vi "Strain Measurement Loop.vi"(6 "Which Program?":T1, 8 "error in":errorcluster, 9 "IBM OptoElectroMechanics Configuration":T2={"Parameter Analizer"={"Parameter Analyzer VISA Session"="COM1", "Sweeping Time Parameters"={"Integration Time"=0, "Short Integration Time (s)"=1.0, "Long Integration Time (s)"=0.0, "Wait Time Parameter"=1.0}, "Acquisition Mode"=enum."Sweeping Mode", "Status Polling Time (ms)"=0, "Comment"="Test VI", "SMU 1 - Sweeping"={"Start / Offset"=0.0, "Stop / Ratio"=1.0, "Step \n(linear only)"=0.01, "Compliance"=0.1, "Power \nCompliance"=0.0, "Mode"=0, "Function"=0, "Sweep Mode"=FALSE}, "SMU 2 - Sweeping"={"Start / Offset"=0.0, "Stop / Ratio"=1.0, "Step \n(linear only)"=0.01, "Compliance"=0.1, "Power \nCompliance"=0.0, "Mode"=0, "Function"=0, "Sweep Mode"=FALSE}, "SMU 3 - Sweeping"={"Start / Offset"=0.0, "Stop / Ratio"=1.0, "Step \n(linear only)"=0.01, "Compliance"=0.1, "Power \nCompliance"=0.0, "Mode"=0, "Function"=0, "Sweep Mode"=FALSE}, "SMU 4 - Sweeping"={"Start / Offset"=0.0, "Stop / Ratio"=1.0, "Step \n(linear only)"=0.01, "Compliance"=0.1, "Power \nCompliance"=0.0, "Mode"=0, "Function"=0, "Sweep Mode"=FALSE}, "Sweep Spacing"=0, "Range"=0, "SMU1 - Sampling"={"Source"=10.0, "Compliance"=1e-05, "Mode"=0, "Function"=FALSE}, "SMU2 - Sampling"={"Source"=1.0, "Compliance"=1.0, "Mode"=0, "Function"=FALSE}, "SMU3 - Sampling"={"Source"=10.0, "Compliance"=1e-05, "Mode"=0, "Function"=FALSE}, "SMU4 - Sampling"={"Source"=0.1, "Compliance"=60.0, "Mode"=10, "Function"=FALSE}, "Sampling Time Parameters"={"Initial Interval (s)"=0.1, "Number of Samples"=60, "Total Sampling Time (s)"=10.0, "Hold Time (s)"=0.0, "Sampling Mode"=0, "Sampling Time"=0}, "Stop Condition"={"Enable Delay (s)"=0.0, "Name"="", "Threshold"=0.0, "num. of events"=1, "Event"=0, "Stop Condition Enable"=FALSE}}, "Switching Matrix"={"Switching Matrix VISA Session"="GPIB0::18::INSTR", "Connections"=[{"Connections"=[FALSE, FALSE, FALSE, FALSE, FALSE, FALSE, FALSE, FALSE, FALSE, FALSE, FALSE, FALSE], "Connection Type"=enum."Disconnected"}, {"Connections"=[FALSE, FALSE, FALSE, FALSE, FALSE, FALSE, FALSE, FALSE, FALSE, FALSE, FALSE, FALSE], "Connection Type"=enum."Disconnected"}, {"Connections"=[FALSE, FALSE, FALSE, FALSE, FALSE, FALSE, FALSE, FALSE, FALSE, FALSE, FALSE, FALSE], "Connection Type"=enum."Disconnected"}, {"Connections"=[FALSE, FALSE, FALSE, FALSE, FALSE, FALSE, FALSE, FALSE, FALSE, FALSE, FALSE, FALSE], "Connection Type"=enum."Disconnected"}, {"Connections"=[FALSE, FALSE, FALSE, FALSE, FALSE, FALSE, FALSE, FALSE, FALSE, FALSE, FALSE, FALSE], "Connection Type"=enum."Disconnected"}, {"Connections"=[FALSE, FALSE, FALSE, FALSE, FALSE, FALSE, FALSE, FALSE, FALSE, FALSE, FALSE, FALSE], "Connection Type"=enum."Disconnected"}, {"Connections"=[FALSE, FALSE, FALSE, FALSE, FALSE, FALSE, FALSE, FALSE, FALSE, FALSE, FALSE, FALSE], "Connection Type"=enum."Disconnected"}, {"Connections"=[FALSE, FALSE, FALSE, FALSE, FALSE, FALSE, FALSE, FALSE, FALSE, FALSE, FALSE, FALSE], "Connection Type"=enum."Disconnected"}]}, "Stress Control"={"Stress Control VISA Session"="StrainMotor", "Axis"=0, "Motion"=0, "Destination (°)"=0.0, "Speed (°/s)"=4.0, "Position (°)"=25.0}, "Optical Spectrometer"={"Laser Settings"={"Laser Wavelength"=enum."365 nm", "Neutral Density Filter"=enum."100%"}, "Spectrometer Settings"={"Confocal Hole Size (µm)"=0.0, "Grating"=2, "Detector"=enum."InGaAs Array"}, "Acquisition Settings"={"Acquisition Mode"=enum."Multi-Window", "Spectal Position (nm)"=632.0, "From (nm)"=735.0, "To (nm)"=0.0, "Integration Time (s)"=0.0, "Number of Accumulations"=3, "AutoScanning"=FALSE, "Spike Removal"=FALSE}, "Path"=path "C:/07 - Prizes and Awards/Marie Curie Prize/Reply Editors Final NCOMMS(10).docx"}, "Switches & Mirrors"={"Relay VISA Session"="COM1", "Switches"={"Laser"=FALSE, "Video"=FALSE}, "Delays (ms)"={"Laser"=500, "Video"=1500}}, "Camera"={"Settings"={"Pixel clock"=20, "Frame rate"=30.0, "Exposure time"=33.21525, "Master Gain"=0, "Red Gain"=0, "Green Gain"=0, "Blue Gain"=0, "Auto Gain"=FALSE, "White-balance"=FALSE, "Color Correction"=FALSE}}, "XYZ Stage"={"Connection Settings"={"Tango VISA"="", "Baudrate"=57600, "Show Protocol?"=FALSE}, "Manual Control"={"North"=FALSE, "South"=FALSE, "West"=FALSE, "East"=FALSE, "Up"=FALSE, "Down"=FALSE, "Stop"=FALSE, "XY Step"=0.0, "Z step"=0.0}, "Coordinate Control"={"Motion Mode"=enum."Absolute", "Destination [mm]"=[]}}, "AutoFocus"={"Matching Criteria"={"Minimum Score"=700.0, "Color Score Weight"=700.0, "Minimum Contrast"=50, "Match Mode"=0, "Match Feature Mode"=0, "Subpixel Accuracy"=TRUE, "Color Sensitivity"=1, "Search Strategy"=1}, "Z Scan Parameters"={"Z Range"=1380.0, "Resolution"=5000.0, "Initial Direction"=enum."Up", "Focus Threshold"=0.1, "Ascent Constant"=0.1}, "Displacement"=0.0, "Transformation Matrix"=[]}, "Sava Data"={"Workspace Info"={"Device Name"="ProberHead_Tst_C29K3_7(2)", "Device Info"="ProberHead_Tst_C29", "Path"=path "C:/Users/gio/Desktop/ProbeHeadTest"}, "Instrument Configuration"={"Instrument"=enum."Unknown Instrument", "Configuration"="Test Configuration"}, "Stress Motor Position"=0.0, "Electrical Measurement"={"Sequence"=[], "V1"=[], "V2"=[], "V3"=[], "V4"=[], "I1"=[], "I2"=[], "I3"=[], "I4"=[]}, "Optical Spectrum"={"Intensity"=[], "Wavelength"=[], "Energy"=[], "Raman Shift"=[], "Detector Temperature"=0.0}}, "PlotData"={"Sliders"={"Strain Sequence"=0, "Instrument Sequence"=0}, "Measurement"={"Which Instrument?"=enum."No Plot", "Electrical Measurement"={"Sequence"=[], "V1"=[], "V2"=[], "V3"=[], "V4"=[], "I1"=[], "I2"=[], "I3"=[], "I4"=[]}, "Measurement Mode"=enum."Sweeping Mode", "Optical Spectrum"={"Intensity"=[], "Wavelength"=[], "Energy"=[], "Raman Shift"=[], "Detector Temperature"=0.0}}, "Instrument Steps"=[], "Strain Points"=[]}, "Instrument Sequence"={"Caller VI"=enum."User"}, "Strain Measurement"={"Stress Sequence "={"Max Motor Position"=1380.0, "# Intermediate Points"=5000, "Initial Direction"=enum."Tension"}, "Track?"=FALSE}} {"AutoFocus"."Displacement" scale=1.0..1000.0; "AutoFocus"."Z Scan Parameters"."Focus Threshold" min=0.0 max=1000.0 step=1.0 format="%#_2f"; "AutoFocus"."Z Scan Parameters"."Ascent Constant" min=0.0 max=1000.0 step=1.0 format="%#_2f"; "AutoFocus"."Z Scan Parameters"."Resolution" min=0.0 max=1.0 step=0.01 format="%_2g"; "AutoFocus"."Z Scan Parameters"."Z Range" format="%_3g"; "AutoFocus"."Matching Criteria"."Match Mode" items=["Shift Invariant", "Rotation Invariant"]; "AutoFocus"."Matching Criteria"."Match Feature Mode" items=["Color and Shape", "Color", "Shape"]; "AutoFocus"."Matching Criteria"."Color Sensitivity" items=["Low Sensitivity", "Medium Sensitivity", "High Sensitivity"]; "AutoFocus"."Matching Criteria"."Search Strategy" items=["Conservative", "Balance", "Aggressive", "Very Aggressive"]; "XYZ Stage"."Manual Control"."Z step" scale=0.1..10.0; "XYZ Stage"."Manual Control"."XY Step" scale=0.1..1000.0; "Camera"."Settings"."Blue Gain" min=0 max=100 scale=0.0..100.0; "Camera"."Settings"."Green Gain" min=0 max=100 scale=0.0..100.0; "Camera"."Settings"."Red Gain" min=0 max=100 scale=0.0..100.0; "Camera"."Settings"."Master Gain" min=0 max=100 scale=0.0..100.0; "Camera"."Settings"."Exposure time" min=0.101625 max=159.246375 step=0.101625 scale=0.101625..159.246375 scale format="%#.3g"; "Camera"."Settings"."Frame rate" min=2.7455631699174137 max=6.2675785993528725 step=0.000101625 scale=2.7455631699174137..6.2675785993528725 scale format="%^#_3g"; "Camera"."Settings"."Pixel clock" min=5 max=43 scale=5.0..43.0; "PlotData"."Sliders"."Instrument Sequence" scale=0.0..10.0; "PlotData"."Sliders"."Strain Sequence" scale=0.0..10.0; "Strain Measurement"."Stress Sequence"."# Intermediate Points" max=1390; "Parameter Analizer"."Stop Condition"."Event" items=["Value > Threshold", "Value < Threshold", "| Value | > | Threshold |", "| Value | < | Threshold |"]; "Parameter Analizer"."Stop Condition"."Threshold" format="%^.2e"; "Parameter Analizer"."Stop Condition"."Enable Delay (s)" format="%.1f"; "Parameter Analizer"."Sampling Time Parameters"."Sampling Time" items=["Auto (linear only)", "No Limit", "Set Limit"]; "Parameter Analizer"."Sampling Time Parameters"."Sampling Mode" items=["Linear", "Log10", "Log25", "Log50", "Thinned Out"]; "Parameter Analizer"."Sampling Time Parameters"."Hold Time (s)" format="%.4f"; "Parameter Analizer"."Sampling Time Parameters"."Total Sampling Time (s)" format="%.1f"; "Parameter Analizer"."Sampling Time Parameters"."Initial Interval (s)" format="%^.3e"; "Parameter Analizer"."SMU 4 - Sweeping"."Function" items=["Disabled", "Var 1", "Var 2", "Var 1'", "Constant"]; "Parameter Analizer"."SMU 4 - Sweeping"."Mode" items=["V", "I", "V pulse", "I  pulse", "Common"]; "Parameter Analizer"."SMU 4 - Sweeping"."Power \nCompliance" format="%^.2e"; "Parameter Analizer"."SMU 4 - Sweeping"."Compliance" format="%^.2e"; "Parameter Analizer"."SMU 4 - Sweeping"."Step \n(linear only)" format="%^.4e"; "Parameter Analizer"."SMU 4 - Sweeping"."Stop / Ratio" format="%^.4e"; "Parameter Analizer"."SMU 4 - Sweeping"."Start / Offset" format="%^.4e"; "Parameter Analizer"."SMU 3 - Sweeping"."Function" items=["Disabled", "Var 1", "Var 2", "Var 1'", "Constant"]; "Parameter Analizer"."SMU 3 - Sweeping"."Mode" items=["V", "I", "V pulse", "I  pulse", "Common"]; "Parameter Analizer"."SMU 3 - Sweeping"."Power \nCompliance" format="%^.2e"; "Parameter Analizer"."SMU 3 - Sweeping"."Compliance" format="%^.2e"; "Parameter Analizer"."SMU 3 - Sweeping"."Step \n(linear only)" format="%^.4e"; "Parameter Analizer"."SMU 3 - Sweeping"."Stop / Ratio" format="%^.4e"; "Parameter Analizer"."SMU 3 - Sweeping"."Start / Offset" format="%^.4e"; "Parameter Analizer"."SMU 2 - Sweeping"."Function" items=["Disabled", "Var 1", "Var 2", "Var 1'", "Constant"]; "Parameter Analizer"."SMU 2 - Sweeping"."Mode" items=["V", "I", "V pulse", "I  pulse", "Common"]; "Parameter Analizer"."SMU 2 - Sweeping"."Power \nCompliance" format="%^.2e"; "Parameter Analizer"."SMU 2 - Sweeping"."Compliance" format="%^.2e"; "Parameter Analizer"."SMU 2 - Sweeping"."Step \n(linear only)" format="%^.4e"; "Parameter Analizer"."SMU 2 - Sweeping"."Stop / Ratio" format="%^.4e"; "Parameter Analizer"."SMU 2 - Sweeping"."Start / Offset" format="%^.4e"; "Parameter Analizer"."SMU 1 - Sweeping"."Function" items=["Disabled", "Var 1", "Var 2", "Var 1'", "Constant"]; "Parameter Analizer"."SMU 1 - Sweeping"."Mode" items=["V", "I", "V pulse", "I  pulse", "Common"]; "Parameter Analizer"."SMU 1 - Sweeping"."Power \nCompliance" format="%^.2e"; "Parameter Analizer"."SMU 1 - Sweeping"."Compliance" format="%^.2e"; "Parameter Analizer"."SMU 1 - Sweeping"."Step \n(linear only)" format="%^.4e"; "Parameter Analizer"."SMU 1 - Sweeping"."Stop / Ratio" format="%^.4e"; "Parameter Analizer"."SMU 1 - Sweeping"."Start / Offset" format="%^.4e"; "Parameter Analizer"."Sweeping Time Parameters"."Long Integration Time (s)" scale=0.02..2.0; "Parameter Analizer"."Sweeping Time Parameters"."Short Integration Time (s)" scale=8e-05..0.00192; "Parameter Analizer"."Sweeping Time Parameters"."Integration Time" items=["Short", "Long"]; "Parameter Analizer"."Sweeping Time Parameters"."Wait Time Parameter" format="%.1f"; "Parameter Analizer"."SMU4 - Sampling"."Mode" items=["V", "I", "Common"]; "Parameter Analizer"."SMU4 - Sampling"."Compliance" format="%^.2e"; "Parameter Analizer"."SMU4 - Sampling"."Source" format="%^.3e"; "Parameter Analizer"."SMU3 - Sampling"."Mode" items=["V", "I", "Common"]; "Parameter Analizer"."SMU3 - Sampling"."Compliance" format="%^.2e"; "Parameter Analizer"."SMU3 - Sampling"."Source" format="%^.3e"; "Parameter Analizer"."SMU2 - Sampling"."Mode" items=["V", "I", "Common"]; "Parameter Analizer"."SMU2 - Sampling"."Compliance" format="%^.2e"; "Parameter Analizer"."SMU2 - Sampling"."Source" format="%^.3e"; "Parameter Analizer"."SMU1 - Sampling"."Mode" items=["V", "I", "Common"]; "Parameter Analizer"."SMU1 - Sampling"."Compliance" format="%^.2e"; "Parameter Analizer"."SMU1 - Sampling"."Source" format="%^.3e"; "Parameter Analizer"."Range" items=["auto", "fixed", "limited"]; "Parameter Analizer"."Sweep Spacing" items=["linear", "log 10", "log 25", "log 50"]; "Stress Control"."Axis" min=1 max=3; "Stress Control"."Position (°)" format="%.6g"; "Stress Control"."Speed (°/s)" min=0.0 max=4.0 format="%.6f"; "Stress Control"."Destination (°)" min=-2000000000.0 max=2000000000.0 format="%.6f"; "Stress Control"."Motion" items=["Absolute", "Relative"]; "Optical Spectrometer"."Spectrometer Settings"."Grating" items=["1800 l/mm", "150 l/mm"]}, 10 "Message Queues out":T58, 11 "Notifiers":T45) -> (0 "error out":errorcluster)   [LabVIEW 2014]
uses:
  support/Message Queue/All Message Queues.ctl
  support/Message Queue/Message Cluster.ctl
  support/Notifiers/Notifiers.ctl
  support/Message Handler Loop Notifiers.ctl
  Hardware Control/Parameter Analyzer/Parameter Analyzer Notifiers.ctl
  Hardware Control/Switching Matrix/Switching Matrix Notifiers.ctl
  Hardware Control/Stress Control/StressControl Notifiers.ctl
  Hardware Control/Spectrometer/Spectrometer Notifiers.ctl
  Hardware Control/Switches and Mirrors/SwitchesMirrors Notifiers.ctl
  Hardware Control/Camera/Camera Notifiers.ctl
  Hardware Control/XYZ Stage/XYZ Notifications.ctl
  Hardware Control/Autofocus/Autofocus Notifiers.ctl
  Measurements/Optoelectronic Measurement/Optoelectronic Notifiers.ctl
  Measurements/Save Data/SaveData Notifiers.ctl
  Measurements/Instrument Sequence/Instrument Sequence Notifiers.ctl
  support/Configuration/Configuration.ctl
  Hardware Control/Parameter Analyzer/Parameter Analyzer Config.ctl
  Hardware Control/Parameter Analyzer/Parameter Analyzer Integration Parameters.ctl
  Hardware Control/Parameter Analyzer/Parameter Analyzer SMU Sweeping.ctl
  Hardware Control/Parameter Analyzer/Parameter Analyzer Sweep Spacing.ctl
  Hardware Control/Parameter Analyzer/Parameter Analyzer SMU Range.ctl
  Hardware Control/Parameter Analyzer/Parameter Analyzer SMU Sampling.ctl
  Hardware Control/Parameter Analyzer/Parameter Analyzer Sampling Parameters.ctl
  Hardware Control/Parameter Analyzer/Parameter Analyzer Stop Sampling Conditions.ctl
  Hardware Control/Switching Matrix/Switching Matrix Config.ctl
  Hardware Control/Stress Control/StressControl Config.ctl
  Hardware Control/Spectrometer/Spectrometer Config.ctl
  Hardware Control/Spectrometer/Laser Settings.ctl
  Hardware Control/Spectrometer/Laser.ctl
  Hardware Control/Spectrometer/Filter.ctl
  Hardware Control/Spectrometer/Grating Detector Settings.ctl
  Hardware Control/Spectrometer/Grating.ctl
  Hardware Control/Spectrometer/Detector.ctl
  Hardware Control/Spectrometer/Acquisition Settings.ctl
  Hardware Control/Switches and Mirrors/SwitchesMirrors Config.ctl
  Hardware Control/Switches and Mirrors/SwitchesMirrors Status.ctl
  Hardware Control/Camera/Camera Config.ctl
  Hardware Control/Camera/Camera Settings.ctl
  Hardware Control/XYZ Stage/XYZ Config.ctl
  Hardware Control/XYZ Stage/XYZ Connection Settings.ctl
  Hardware Control/XYZ Stage/XYZ Stage Control.ctl
  Hardware Control/XYZ Stage/XYZ Coordinate Control.ctl
  Hardware Control/Autofocus/AutoFocus Config.ctl
  Hardware Control/Autofocus/ZScan.ctl
  <vilib>/Analysis/Matrix/Datatypes/RealMatrix.ctl
  Measurements/Save Data/SaveData Config.ctl
  Measurements/Save Data/SaveData Workspace Info.ctl
  Measurements/Save Data/SaveData Instrument Configuration.ctl
  Measurements/Instrument Sequence/Instrument List.ctl
  Hardware Control/Spectrometer/Spectral Data.ctl
  Measurements/Plot Data/PlotData Config.ctl
  Measurements/Plot Data/Measurement.ctl
  Measurements/Plot Data/WhichInstrument.ctl
  Hardware Control/Parameter Analyzer/Electrical Data.ctl
  Measurements/Instrument Sequence/Instrument Steps.ctl
  Measurements/Instrument Sequence/Action.ctl
  Measurements/Instrument Sequence/Instrument Sequence Config.ctl
  Measurements/Strain Measurement/Strain Measurement Config.ctl
  Measurements/Instrument Sequence/Instrument Stequence - Which Program.ctl
  Measurements/Strain Measurement/Strain Measurement Function.ctl
  support/Message Queue/Message Queue.lvlib
  <vilib>/Analysis/Matrix/NI_Matrix.lvlib
panel:
  # "LICENSED MATERIALS – PROPERTY OF IBM\nCopyright IBM Corp. 2016,\nALL RIGHTS RESERVED"
  # "XY"
  # "Z"
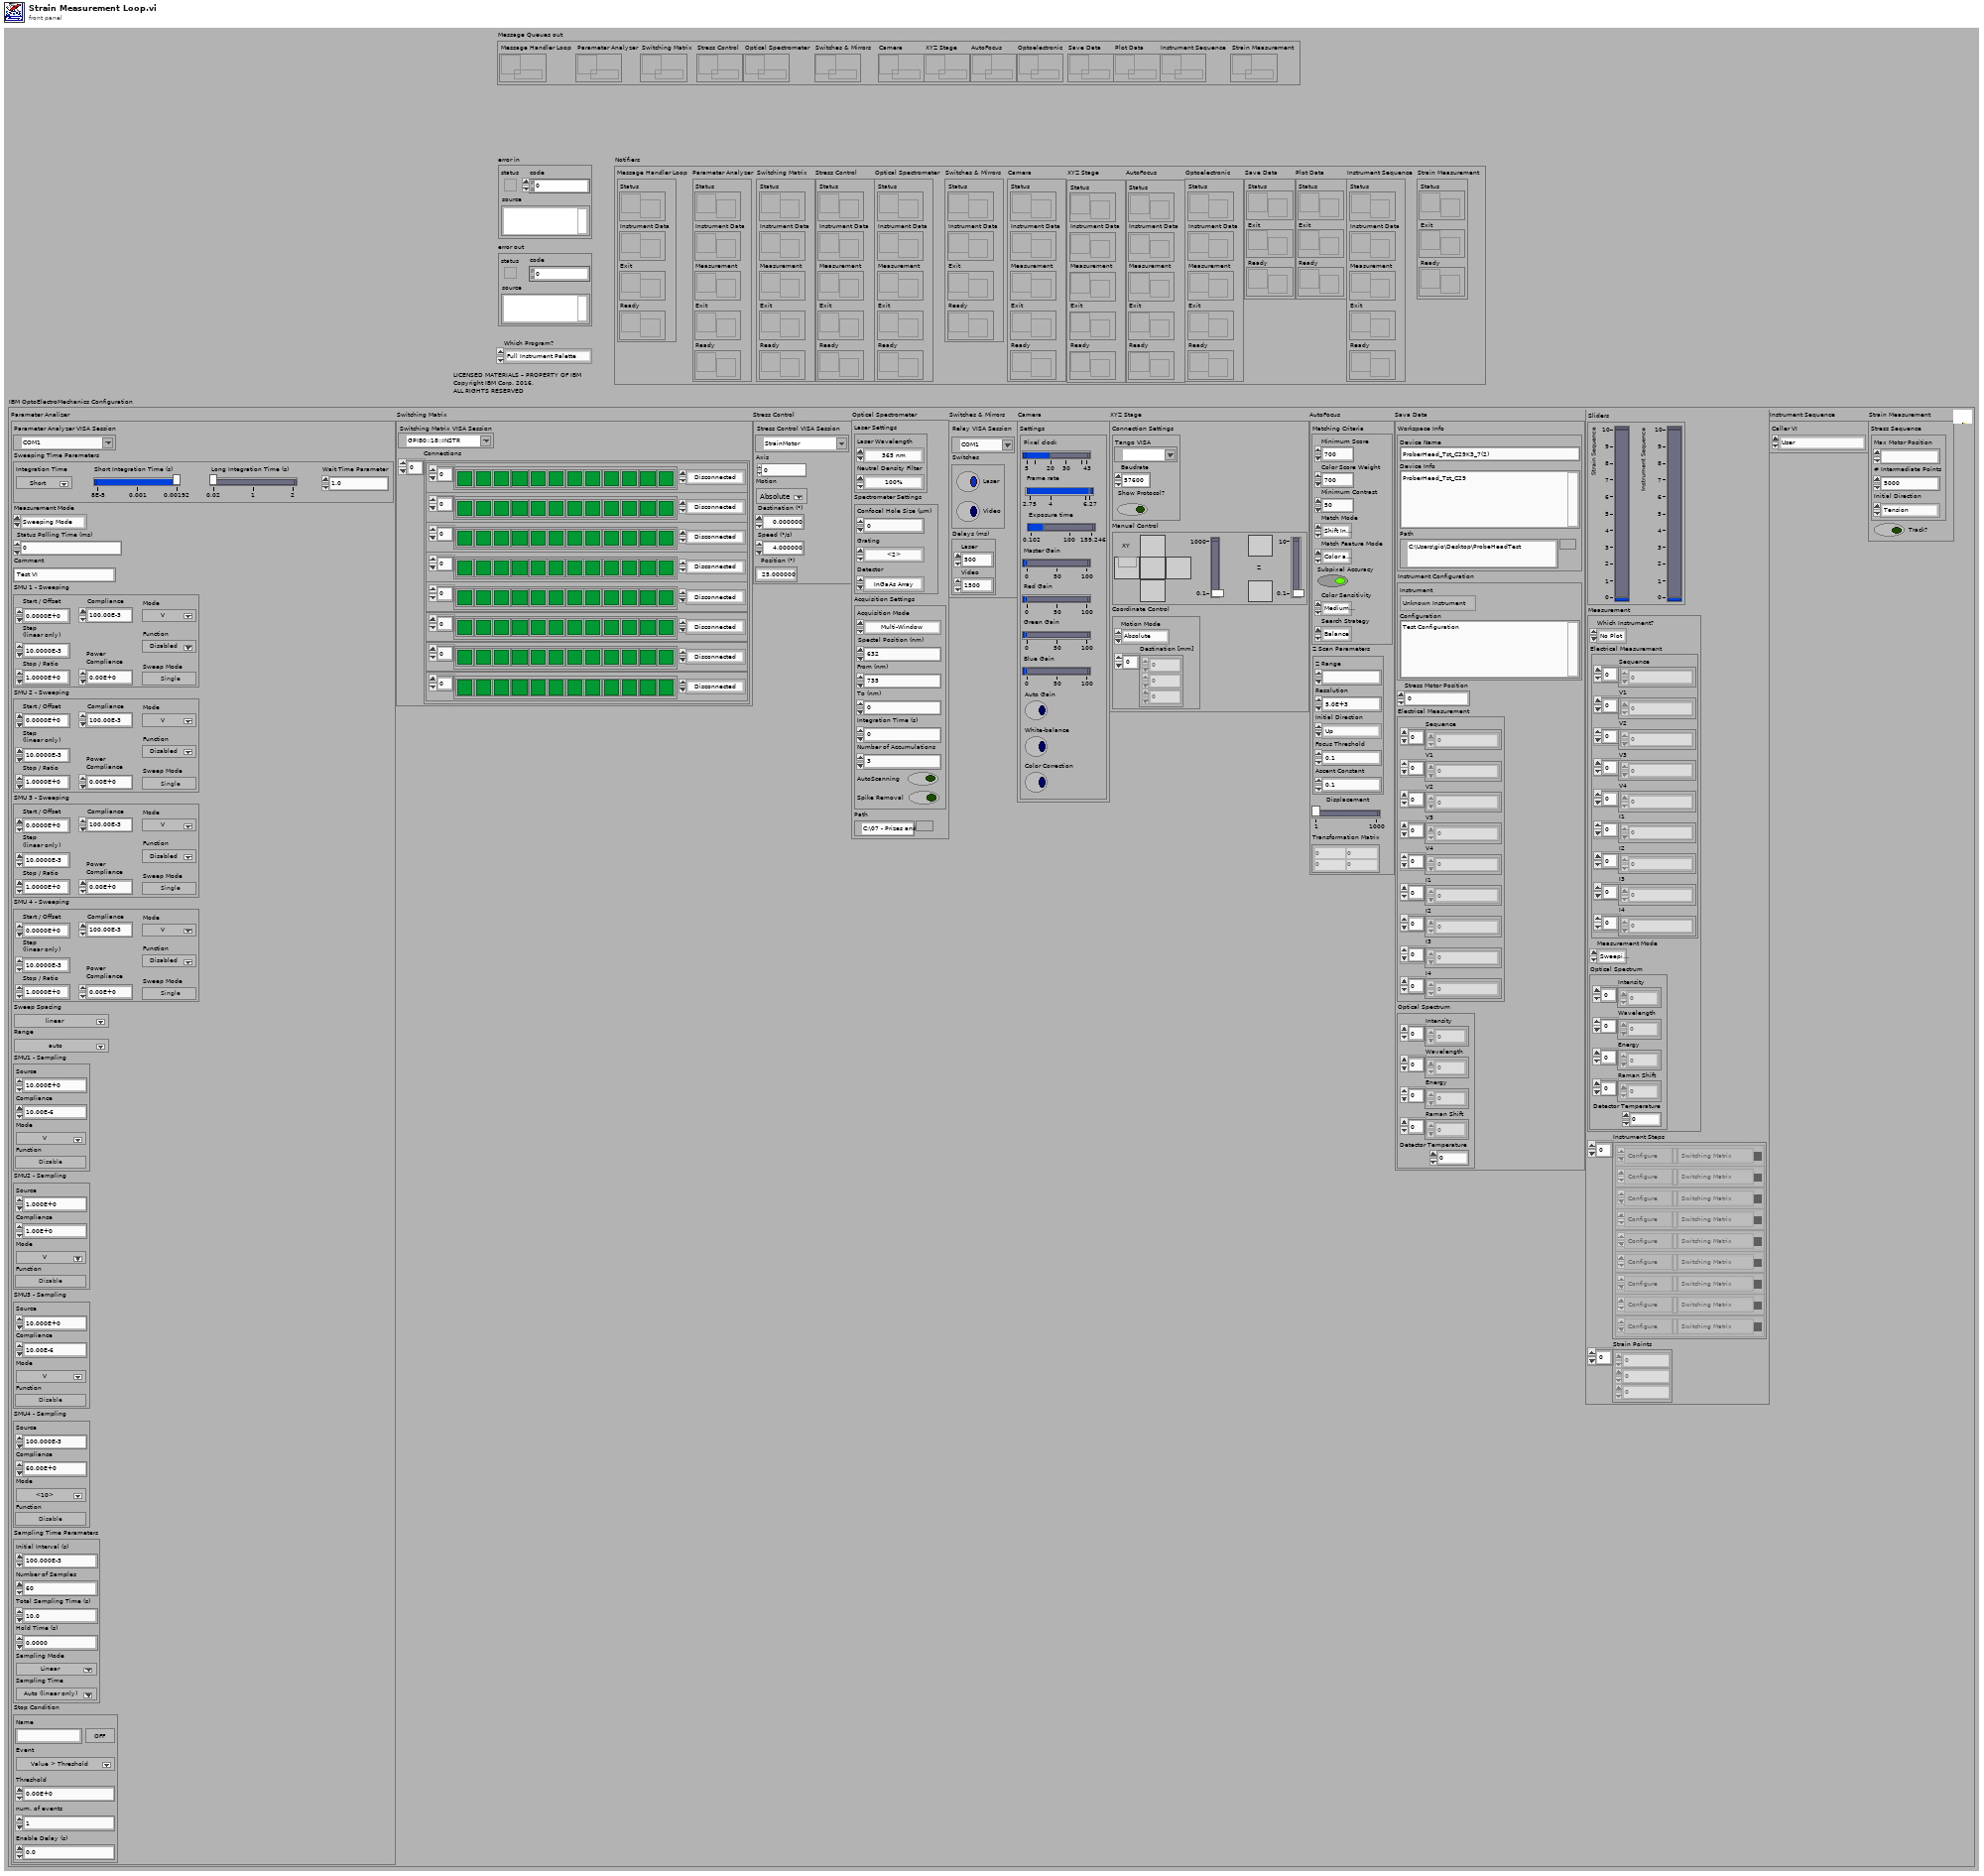
[diagram p1: front panel]
types:
  T1 = typedef "Instrument Stequence - Which Program.ctl" = enum16{"Full Instrument Palette", "Strain Electrical"}
  T2 = typedef "Configuration.ctl" = cluster{"Parameter Analizer":T3, "Switching Matrix":T11, "Stress Control":T12, "Optical Spectrometer":T13, "Switches & Mirrors":T21, "Camera":T23, "XYZ Stage":T25, "AutoFocus":T29, "Sava Data":T32, "PlotData":T37, "Instrument Sequence":T43, "Strain Measurement":T44}
  T3 = typedef "Parameter Analyzer Config.ctl" = cluster{"Parameter Analyzer VISA Session":refnum<visa-resource-name>, "Sweeping Time Parameters":T4, "Acquisition Mode":enum32{"Sweeping Mode", "Sampling Mode"}, "Status Polling Time (ms)":u32, "Comment":string, "SMU 1 - Sweeping":T5, "SMU 2 - Sweeping":T5, "SMU 3 - Sweeping":T5, "SMU 4 - Sweeping":T5, "Sweep Spacing":T6, "Range":T7, "SMU1 - Sampling":T8, "SMU2 - Sampling":T8, "SMU3 - Sampling":T8, "SMU4 - Sampling":T8, "Sampling Time Parameters":T9, "Stop Condition":T10}
  T4 = typedef "Parameter Analyzer Integration Parameters.ctl" = cluster{"Integration Time":u32, "Short Integration Time (s)":dbl, "Long Integration Time (s)":dbl, "Wait Time Parameter":dbl}
  T5 = typedef "Parameter Analyzer SMU Sweeping.ctl" = cluster{"Start / Offset":dbl, "Stop / Ratio":dbl, "Step \n(linear only)":dbl, "Compliance":dbl, "Power \nCompliance":dbl, "Mode":u32, "Function":i32, "Sweep Mode":bool}
  T6 = typedef "Parameter Analyzer Sweep Spacing.ctl" = u16
  T7 = typedef "Parameter Analyzer SMU Range.ctl" = u16
  T8 = typedef "Parameter Analyzer SMU Sampling.ctl" = cluster{"Source":dbl, "Compliance":dbl, "Mode":u32, "Function":bool}
  T9 = typedef "Parameter Analyzer Sampling Parameters.ctl" = cluster{"Initial Interval (s)":dbl, "Number of Samples":i32, "Total Sampling Time (s)":dbl, "Hold Time (s)":dbl, "Sampling Mode":i32, "Sampling Time":i32}
  T10 = typedef "Parameter Analyzer Stop Sampling Conditions.ctl" = cluster{"Enable Delay (s)":dbl, "Name":string, "Threshold":dbl, "num. of events":i32, "Event":i32, "Stop Condition Enable":bool}
  T11 = typedef "Switching Matrix Config.ctl" = cluster{"Switching Matrix VISA Session":refnum<visa-resource-name>, "Connections":cluster{"Connections":bool[], "Connection Type":enum16{"Disconnected", "Make - Break", "Break - Make"}}[]}
  T12 = typedef "StressControl Config.ctl" = cluster{"Stress Control VISA Session":refnum<visa-resource-name>, "Axis":i32, "Motion":u16, "Destination (°)":dbl, "Speed (°/s)":dbl, "Position (°)":dbl}
  T13 = typedef "Spectrometer Config.ctl" = cluster{"Laser Settings":T14, "Spectrometer Settings":T17, "Acquisition Settings":T20, "Path":path}
  T14 = typedef "Laser Settings.ctl" = cluster{"Laser Wavelength":T15, "Neutral Density Filter":T16}
  T15 = typedef "Laser.ctl" = enum16{"633 nm", "784 nm", "532 nm", "365 nm"}
  T16 = typedef "Filter.ctl" = enum16{"100%", "50%", "25%", "10%", "1%", "0.1%", "0.01%"}
  T17 = typedef "Grating Detector Settings.ctl" = cluster{"Confocal Hole Size (µm)":dbl, "Grating":T18, "Detector":T19}
  T18 = typedef "Grating.ctl" = u16
  T19 = typedef "Detector.ctl" = enum16{"InGaAs Array", "Silicon CCD"}
  T20 = typedef "Acquisition Settings.ctl" = cluster{"Acquisition Mode":enum16{"Single Window", "Multi-Window"}, "Spectal Position (nm)":dbl, "From (nm)":dbl, "To (nm)":dbl, "Integration Time (s)":dbl, "Number of Accumulations":i32, "AutoScanning":bool, "Spike Removal":bool}
  T21 = typedef "SwitchesMirrors Config.ctl" = cluster{"Relay VISA Session":refnum<visa-resource-name>, "Switches":T22, "Delays (ms)":cluster{"Laser":u32, "Video":u32}}
  T22 = typedef "SwitchesMirrors Status.ctl" = cluster{"Laser":bool, "Video":bool}
  T23 = typedef "Camera Config.ctl" = cluster{"Settings":T24}
  T24 = typedef "Camera Settings.ctl" = cluster{"Pixel clock":i32, "Frame rate":dbl, "Exposure time":dbl, "Master Gain":i32, "Red Gain":i32, "Green Gain":i32, "Blue Gain":i32, "Auto Gain":bool, "White-balance":bool, "Color Correction":bool}
  T25 = typedef "XYZ Config.ctl" = cluster{"Connection Settings":T26, "Manual Control":T27, "Coordinate Control":T28}
  T26 = typedef "XYZ Connection Settings.ctl" = cluster{"Tango VISA":refnum<visa-resource-name>, "Baudrate":i32, "Show Protocol?":bool}
  T27 = typedef "XYZ Stage Control.ctl" = cluster{"North":bool, "South":bool, "West":bool, "East":bool, "Up":bool, "Down":bool, "Stop":bool, "XY Step":dbl, "Z step":dbl}
  T28 = typedef "XYZ Coordinate Control.ctl" = cluster{"Motion Mode":enum16{"Absolute", "Relative"}, "Destination [mm]":dbl[]}
  T29 = typedef "AutoFocus Config.ctl" = cluster{"Matching Criteria":cluster{"Minimum Score":sgl, "Color Score Weight":sgl, "Minimum Contrast":i32, "Match Mode":u32, "Match Feature Mode":u32, "Subpixel Accuracy":bool, "Color Sensitivity":u32, "Search Strategy":u32}, "Z Scan Parameters":T30, "Displacement":dbl, "Transformation Matrix":T31}
  T30 = typedef "ZScan.ctl" = cluster{"Z Range":ext, "Resolution":dbl, "Initial Direction":enum16{"Up", "Down"}, "Focus Threshold":dbl, "Ascent Constant":dbl}
  T31 = typedef "NI_Matrix.lvlib/RealMatrix.ctl" = dbl[][]
  T32 = typedef "SaveData Config.ctl" = cluster{"Workspace Info":T33, "Instrument Configuration":T34, "Stress Motor Position":dbl, "Electrical Measurement":cluster{"Sequence":dbl[], "V1":dbl[], "V2":dbl[], "V3":dbl[], "V4":dbl[], "I1":dbl[], "I2":dbl[], "I3":dbl[], "I4":dbl[]}, "Optical Spectrum":T36}
  T33 = typedef "SaveData Workspace Info.ctl" = cluster{"Device Name":string, "Device Info":string, "Path":path}
  T34 = typedef "SaveData Instrument Configuration.ctl" = cluster{"Instrument":T35, "Configuration":string}
  T35 = typedef "Instrument List.ctl" = enum32{"Unknown Instrument", "Switching Matrix", "Parameter Analyzer", "Optical Spectrometer", "Optoelectronic", "Autofocus"}
  T36 = typedef "Spectral Data.ctl" = cluster{"Intensity":dbl[], "Wavelength":dbl[], "Energy":dbl[], "Raman Shift":dbl[], "Detector Temperature":dbl}
  T37 = typedef "PlotData Config.ctl" = cluster{"Sliders":cluster{"Strain Sequence":i32, "Instrument Sequence":i32}, "Measurement":T38, "Instrument Steps":T41, "Strain Points":dbl[]}
  T38 = typedef "Measurement.ctl" = cluster{"Which Instrument?":T39, "Electrical Measurement":T40, "Measurement Mode":enum16{"Sweeping Mode", "Sampling Mode"}, "Optical Spectrum":T36}
  T39 = typedef "WhichInstrument.ctl" = enum16{"No Plot", "Spectrometer", "Parameter Analyzer", "Optoelectronic"}
  T40 = typedef "Electrical Data.ctl" = cluster{"Sequence":dbl[], "V1":dbl[], "V2":dbl[], "V3":dbl[], "V4":dbl[], "I1":dbl[], "I2":dbl[], "I3":dbl[], "I4":dbl[]}
  T41 = typedef "Instrument Steps.ctl" = cluster{"Action":T42, "Configuration":variant, "Instrument":T35, "Status":enum8{"False", "True", "Mixed"}}[]
  T42 = typedef "Action.ctl" = enum32{"Configure", "Measure"}
  T43 = typedef "Instrument Sequence Config.ctl" = cluster{"Caller VI":enum16{"User", "Stress Measurement VI"}}
  T44 = typedef "Strain Measurement Config.ctl" = cluster{"Stress Sequence ":cluster{"Max Motor Position":ext, "# Intermediate Points":u32, "Initial Direction":enum16{"Tension", "Compression"}}, "Track?":bool}
  T45 = typedef "Notifiers.ctl" = cluster{"Message Handler Loop":T46, "Parameter Analyzer":T47, "Switching Matrix":T48, "Stress Control":T49, "Optical Spectrometer":T50, "Switches & Mirrors":T51, "Camera":T52, "XYZ Stage":T53, "AutoFocus":T54, "Optoelectronic":T55, "Save Data":T56, "Plot Data":T56, "Instrument Sequence":T57, "Strain Measurement":cluster{"Status":refnum<notifier>, "Exit":refnum<notifier>, "Ready":refnum<notifier>}}
  T46 = typedef "Message Handler Loop Notifiers.ctl" = cluster{"Status":refnum<notifier>, "Instrument Data":refnum<notifier>, "Exit":refnum<notifier>, "Ready":refnum<notifier>}
  T47 = typedef "Parameter Analyzer Notifiers.ctl" = cluster{"Status":refnum<notifier>, "Instrument Data":refnum<notifier>, "Measurement":refnum<notifier>, "Exit":refnum<notifier>, "Ready":refnum<notifier>}
  T48 = typedef "Switching Matrix Notifiers.ctl" = cluster{"Status":refnum<notifier>, "Instrument Data":refnum<notifier>, "Measurement":refnum<notifier>, "Exit":refnum<notifier>, "Ready":refnum<notifier>}
  T49 = typedef "StressControl Notifiers.ctl" = cluster{"Status":refnum<notifier>, "Instrument Data":refnum<notifier>, "Measurement":refnum<notifier>, "Exit":refnum<notifier>, "Ready":refnum<notifier>}
  T50 = typedef "Spectrometer Notifiers.ctl" = cluster{"Status":refnum<notifier>, "Instrument Data":refnum<notifier>, "Measurement":refnum<notifier>, "Exit":refnum<notifier>, "Ready":refnum<notifier>}
  T51 = typedef "SwitchesMirrors Notifiers.ctl" = cluster{"Status":refnum<notifier>, "Instrument Data":refnum<notifier>, "Exit":refnum<notifier>, "Ready":refnum<notifier>}
  T52 = typedef "Camera Notifiers.ctl" = cluster{"Status":refnum<notifier>, "Instrument Data":refnum<notifier>, "Measurement":refnum<notifier>, "Exit":refnum<notifier>, "Ready":refnum<notifier>}
  T53 = typedef "XYZ Notifications.ctl" = cluster{"Status":refnum<notifier>, "Instrument Data":refnum<notifier>, "Measurement":refnum<notifier>, "Exit":refnum<notifier>, "Ready":refnum<notifier>}
  T54 = typedef "Autofocus Notifiers.ctl" = cluster{"Status":refnum<notifier>, "Instrument Data":refnum<notifier>, "Measurement":refnum<notifier>, "Exit":refnum<notifier>, "Ready":refnum<notifier>}
  T55 = typedef "Optoelectronic Notifiers.ctl" = cluster{"Status":refnum<notifier>, "Instrument Data":refnum<notifier>, "Measurement":refnum<notifier>, "Exit":refnum<notifier>, "Ready":refnum<notifier>}
  T56 = typedef "SaveData Notifiers.ctl" = cluster{"Status":refnum<notifier>, "Exit":refnum<notifier>, "Ready":refnum<notifier>}
  T57 = typedef "Instrument Sequence Notifiers.ctl" = cluster{"Status":refnum<notifier>, "Instrument Data":refnum<notifier>, "Measurement":refnum<notifier>, "Exit":refnum<notifier>, "Ready":refnum<notifier>}
  T58 = typedef "Message Queue.lvlib/All Message Queues.ctl" = cluster{"Message Handler Loop":refnum<queue>, "Parameter Analyzer":refnum<queue>, "Switching Matrix":refnum<queue>, "Stress Control":refnum<queue>, "Optical Spectrometer":refnum<queue>, "Switches & Mirrors":refnum<queue>, "Camera":refnum<queue>, "XYZ Stage":refnum<queue>, "AutoFocus":refnum<queue>, "Optoelectronic":refnum<queue>, "Save Data":refnum<queue>, "Plot Data":refnum<queue>, "Instrument Sequence":refnum<queue>, "Strain Measurement":refnum<queue>}
  T59 = typedef "Strain Measurement Data.ctl" = cluster{"Configuration":T44, "Refnums":T60}
  T60 = typedef "Strain Measurement Refnums.ctl" = cluster{"Instrument Steps":refnum<vi>, "Sequence Progress":refnum<vi>, "Device ID":refnum<vi>, "Device Information":refnum<vi>, "Pause-Resume":refnum<vi>, "Track":refnum<vi>, "Plot":T61}
  T61 = typedef "Electrical Data Plot Refnums.ctl" = cluster{"Plot List":refnum<vi>, "Voltage Plot":refnum<vi>, "Current Plot":refnum<vi>, "IV Characteristic":refnum<vi>, "dI/dV-V Characteristic":refnum<vi>}
  T62 = typedef "Strain Measurement Function.ctl" = enum16{"Get Stress Controller Status", "Define Strain Sequence", "Update Track", "Decide on Track", "Reset Strain Sequence", "Start Strain Measurement", "Set Strain Sequence Step", "Add Instrument Sequence Step", "Delete Instrument Sequence Step", "Clear Instrument Sequence", "Reset Instrument Sequence", "Load Instrument Sequence", "Save Instrument Sequence", "Measure Instrument Sequence", "Choose What Next", "Configure Stress Control", "Set Workspace Data", "Save to Workspace", "Update Sequence Status", "Pause", "Stop", "Update Refnums"}
  T63 = cluster{"Max Motor Position":ext, "# Intermediate Points":u32, "Initial Direction":enum16{"Tension", "Compression"}}
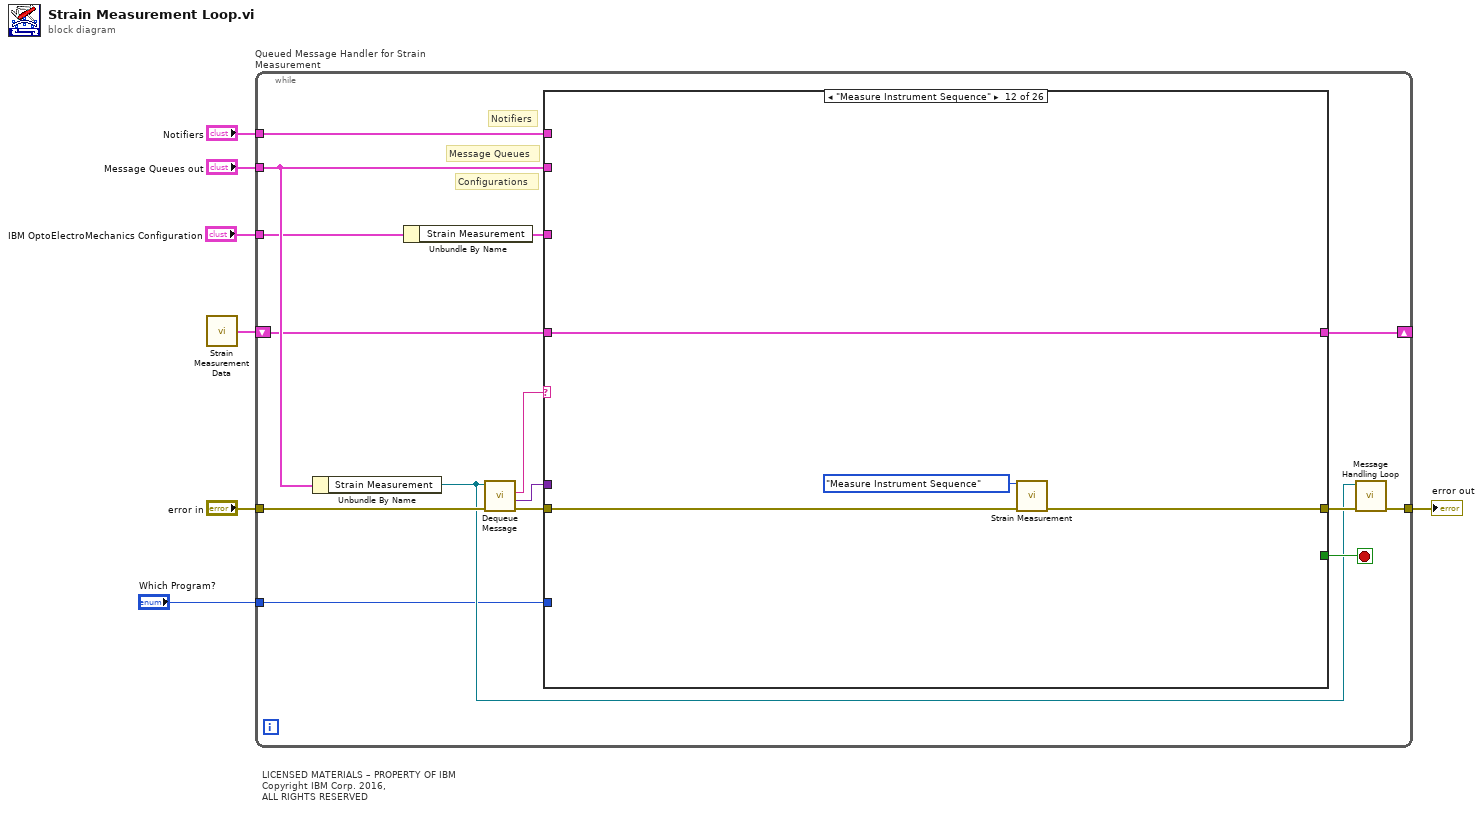
[diagram p0: block diagram]
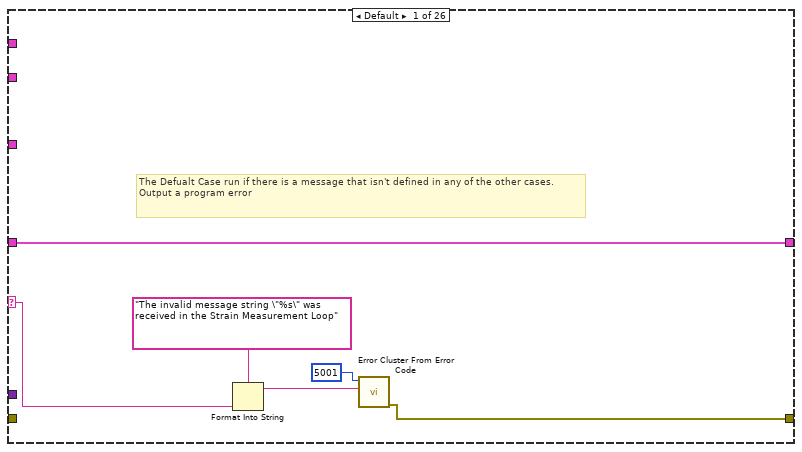
[diagram p2: hidden frame]
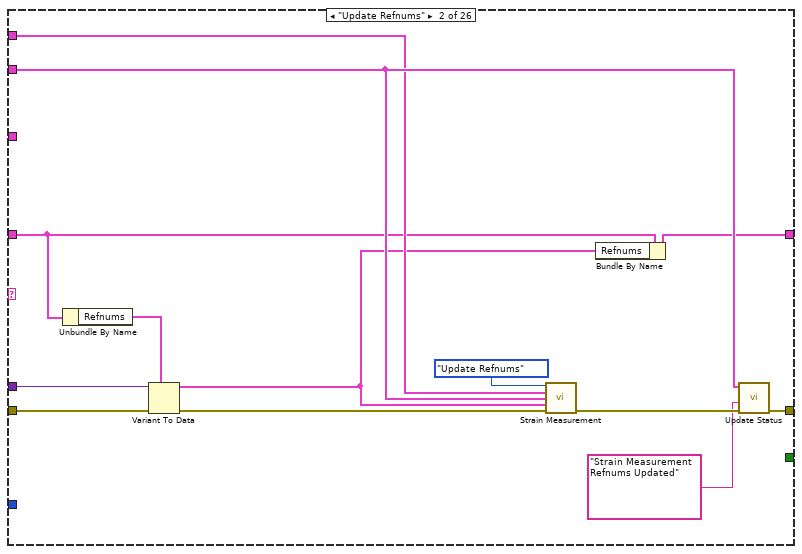
[diagram p3: hidden frame]
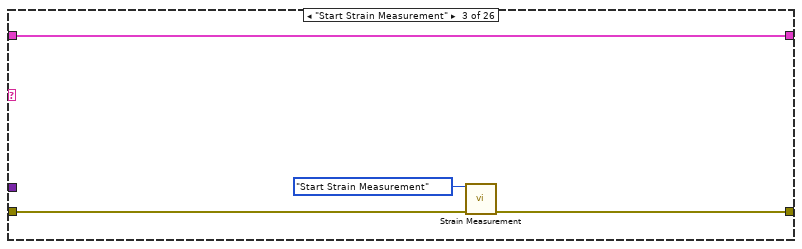
[diagram p4: hidden frame]
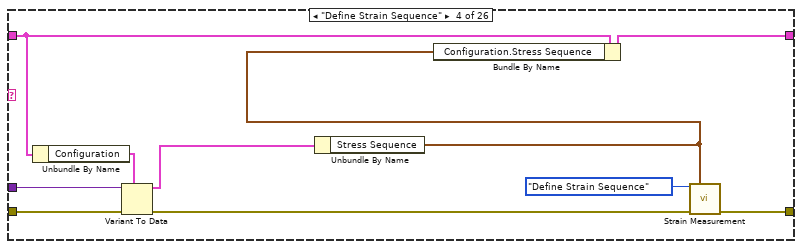
[diagram p5: hidden frame]
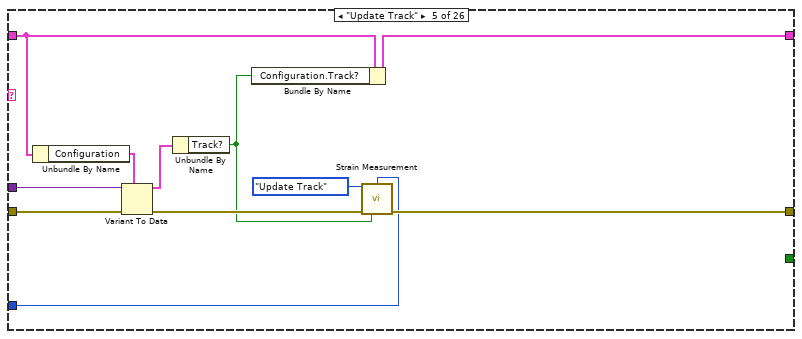
[diagram p6: hidden frame]
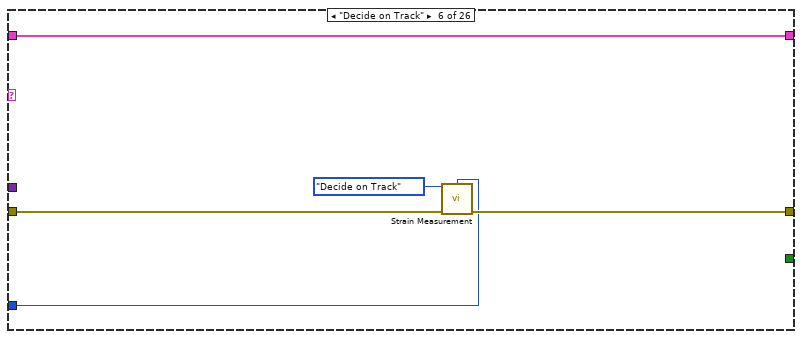
[diagram p7: hidden frame]
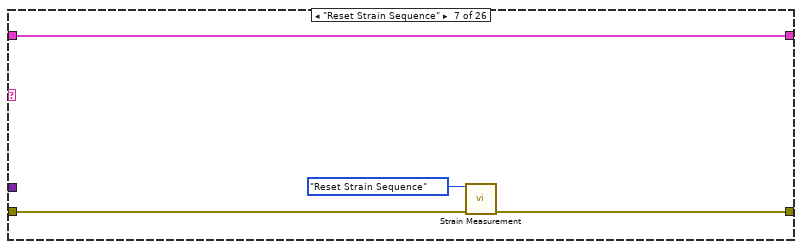
[diagram p8: hidden frame]
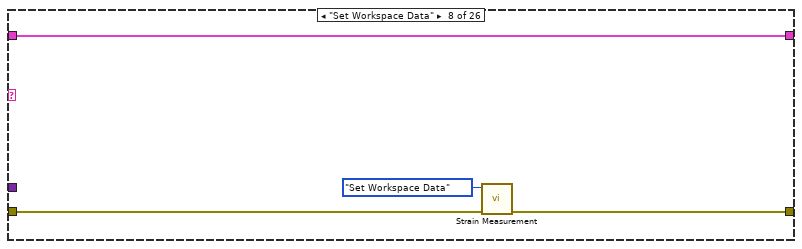
[diagram p9: hidden frame]
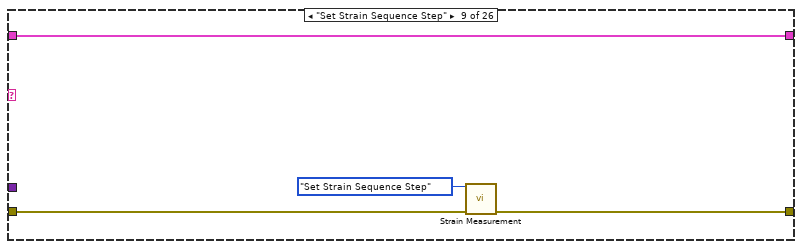
[diagram p10: hidden frame]
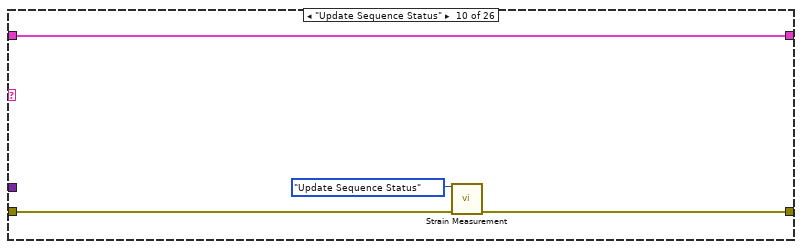
[diagram p11: hidden frame]
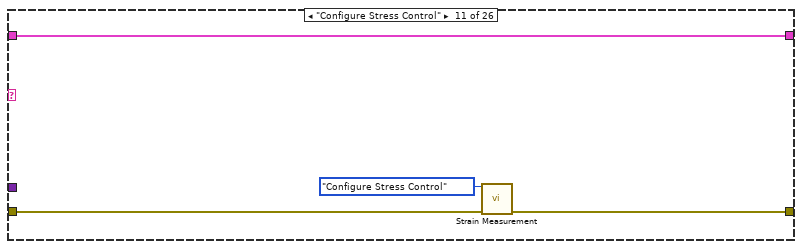
[diagram p12: hidden frame]
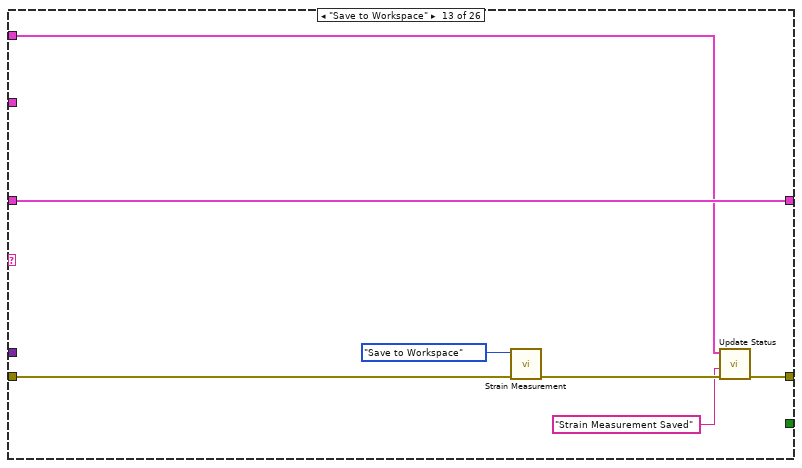
[diagram p13: hidden frame]
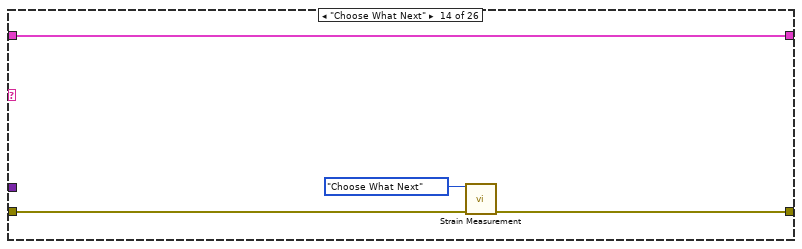
[diagram p14: hidden frame]
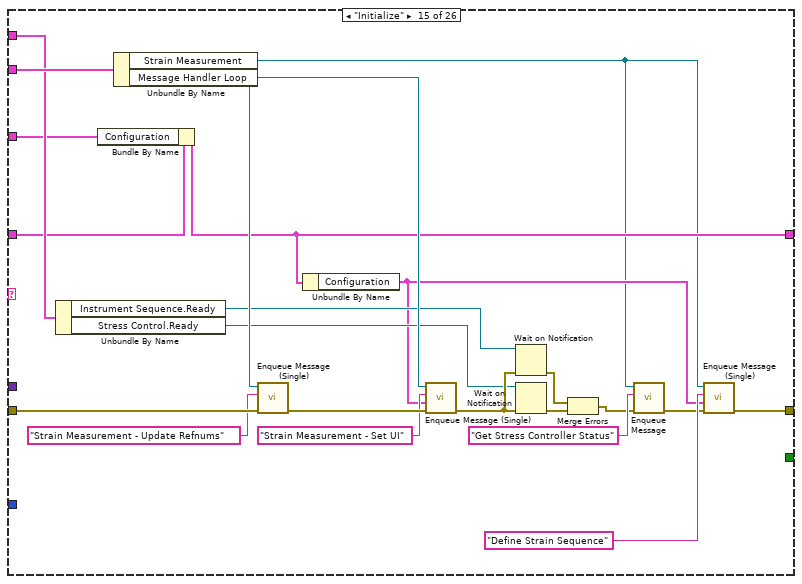
[diagram p15: hidden frame]
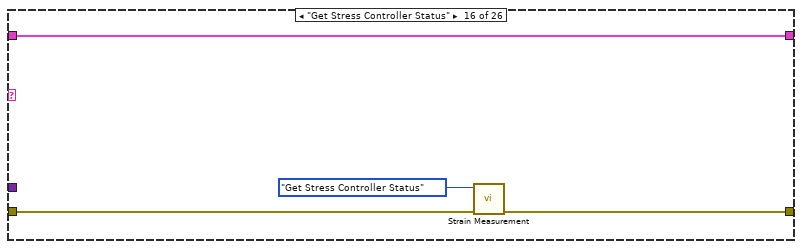
[diagram p16: hidden frame]
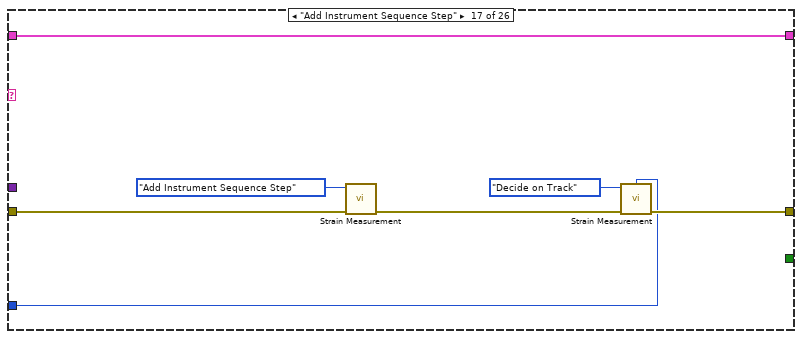
[diagram p17: hidden frame]
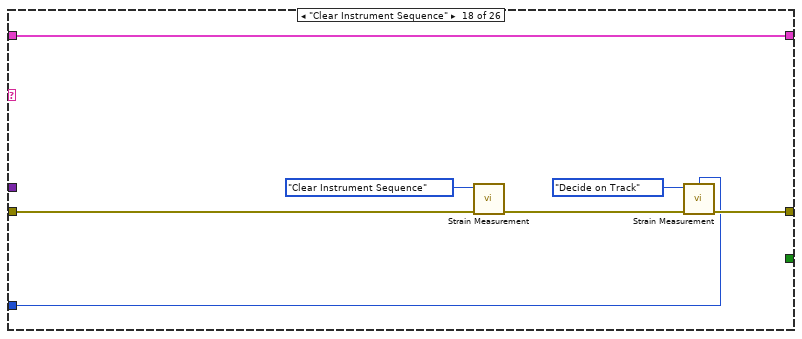
[diagram p18: hidden frame]
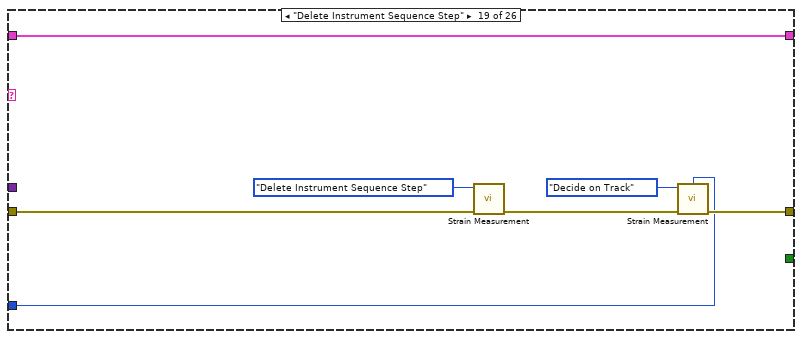
[diagram p19: hidden frame]
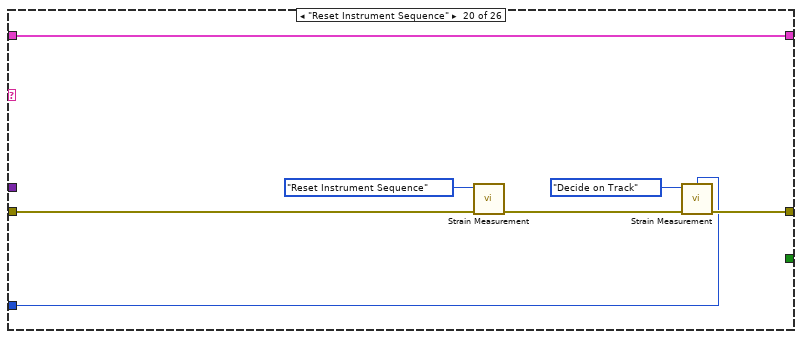
[diagram p20: hidden frame]
diagram:
  # "LICENSED MATERIALS – PROPERTY OF IBM\nCopyright IBM Corp. 2016,\nALL RIGHTS RESERVED"
  n1 = call "Strain Measurement Data.vi"() -> ("Strain-Electrical Measurement"=w3:T59)
  n2 = while "Queued Message Handler for Strain Measurement" {
    tunnel: "error in" -> [w22]
    tunnel: [w14] -> w4
    tunnel: "Message Queues out" -> [w18]
    tunnel: "Notifiers" -> [w17]
    shift-right: [w11] -> _
    shift-left: w3 -> [w12]
    tunnel: "IBM OptoElectroMechanics Configuration" -> [w10]
    tunnel: "Which Program?" -> [w8]
    stop <- w16 stop-if-true
    # "Configurations"
    # "Notifiers"
    # "Message Queues"
    n3 = Unbundle By Name(w18) -> ("Strain Measurement"=w13:refnum<queue>)
    n4 = Unbundle By Name(w10) -> ("Strain Measurement"=w9:T44)
    n5 = call "Dequeue Message.vi"("error in (no error)"=w22, "Message Queue"=w13) -> ("error out"=w21:errorcluster, "Message Data"=w19:variant, "Message"=w20:string)  [unwired: 7 out]
    n6 = case shown="\"Measure Instrument Sequence\"" w20 {
      selector: w20 -> [w25 _ _ _ _ _ _ _ _ _ _ _ _ _ _ _ _ _ _ _ _ _ _ _ _ _]
      tunnel: w21 -> [_ w40 w44 w55 w66 w68 w72 w76 w82 w87 w91 w95 w102 w105 w126 w132 w139 w146 w153 w160 w167 w171 w175 w182 w191 w206]
      tunnel: [w24 w39 w42 w52 w63 w71 w75 w79 w80 w86 w90 w94 w98 w106 w121 w131 w134 w141 w149 w155 w162 w170 w174 w178 w186 w200] -> w15
      tunnel: w19 -> [_ w41 _ w54 w65 _ _ _ _ _ _ _ _ _ _ _ _ _ _ _ _ _ _ _ w184 _]
      tunnel: w18 -> [_ w35 _ _ _ _ _ _ _ _ _ _ w100 _ w128 _ _ _ _ _ _ _ _ w176 w192 w209]
      tunnel: w17 -> [_ w34 _ _ _ _ _ _ _ _ _ _ _ _ w127 _ _ _ _ _ _ _ _ _ _ w201]
      tunnel: [_ _ _ _ _ _ _ _ _ _ _ _ _ _ _ _ _ _ _ _ _ _ _ _ _ TRUE ("Priority Message? (F)")] -> w16
      tunnel: w12 -> [w23 w32 w43 w48 w60 w69 w73 w77 w81 w85 w89 w93 w101 w104 w114 w130 w138 w145 w152 w159 w166 w169 w173 w181 w183 w207]
      tunnel: [w23 w33 w43 w50 w61 w69 w73 w77 w81 w85 w89 w93 w101 w104 w113 w130 w138 w145 w152 w159 w166 w169 w173 w181 w183 w207] -> w11
      tunnel: w9 -> [_ _ _ _ _ _ _ _ _ _ _ _ _ _ w112 _ _ _ _ _ _ _ _ _ _ _]
      tunnel: w8 -> [_ _ _ _ w56 w67 _ _ _ _ _ _ _ _ _ _ w133 w140 w147 w154 w161 _ _ _ _ _]
      frame Default {
        # "The Defualt Case run if there is a message that isn't defined in any of the other cases.\nOutput a program error"
        n7 = Format Into String(format string="The invalid message string \"%s\" was  received in the Strain Measurement Loop", w25) -> (resulting string=w27:string)  [unwired: 2 in, 1 out]
        n8 = call <vilib>:"Error Cluster From Error Code.vi"("error message (\"\")"=w27, "error code (0)"=5001) -> ("error out"=w24:errorcluster)  [unwired: 2 in, 5 out]
      }
      frame "Update Refnums" {
        n9 = Unbundle By Name(w32) -> ("Refnums"=w31:T60)
        n10 = Variant To Data(error in=w40, type=w31, Variant=w41) -> (data=w30:T60, error out=w36:errorcluster)
        n11 = call "Strain Measurement.vi"("Function"=Strain_Measurement_Function."Update Refnums", "Notifiers"=w34, "Message Queues"=w35, "Refnums"=w30, "error in (no error)"=w36) -> ("error out"=w38:errorcluster)  [unwired: 3 in, 7 out]
        n12 = Bundle By Name(cluster=w32, "Refnums"=w30) -> (w33:T59)
        n13 = call "Update Status.vi"("error in"=w38, "String"="Strain Measurement Refnums Updated" ("button name (\"OK\")"), "Message Queues out"=w35) -> ("error out"=w39:errorcluster)  [unwired: 8 out]
      }
      frame "Start Strain Measurement" {
        n14 = call "Strain Measurement.vi"("Function"=Strain_Measurement_Function."Start Strain Measurement", "error in (no error)"=w44) -> ("error out"=w42:errorcluster)  [unwired: 6 in, 7 out]
      }
      frame "Define Strain Sequence" {
        n15 = Unbundle By Name(w48) -> ("Configuration"=w47:T44)
        n16 = Variant To Data(error in=w55, type=w47, Variant=w54) -> (data=w51:T44, error out=w53:errorcluster)
        n17 = Unbundle By Name(w51) -> ("Stress Sequence"=w49:T63)
        n18 = Bundle By Name(cluster=w48, "Configuration.Stress Sequence"=w49) -> (w50:T59)
        n19 = call "Strain Measurement.vi"("Function"=Strain_Measurement_Function."Define Strain Sequence", "Stress Sequence Parameters"=w49, "error in (no error)"=w53) -> ("error out"=w52:errorcluster)  [unwired: 5 in, 7 out]
      }
      frame "Update Track" {
        n20 = Unbundle By Name(w60) -> ("Configuration"=w59:T44)
        n21 = Variant To Data(error in=w66, type=w59, Variant=w65) -> (data=w62:T44, error out=w64:errorcluster)
        n22 = Unbundle By Name(w62) -> ("Track?"=w57:bool)
        n23 = Bundle By Name(cluster=w60, "Configuration.Track?"=w57) -> (w61:T59)
        n24 = call "Strain Measurement.vi"("Function"=Strain_Measurement_Function."Update Track", "Which Program?"=w56, "error in (no error)"=w64, "Track"=w57) -> ("error out"=w63:errorcluster)  [unwired: 4 in, 7 out]
      }
      frame "Decide on Track" {
        n25 = call "Strain Measurement.vi"("Function"=Strain_Measurement_Function."Decide on Track", "Which Program?"=w67, "error in (no error)"=w68) -> ("error out"=w71:errorcluster)  [unwired: 5 in, 7 out]
      }
      frame "Reset Strain Sequence" {
        n26 = call "Strain Measurement.vi"("Function"=Strain_Measurement_Function."Reset Strain Sequence", "error in (no error)"=w72) -> ("error out"=w75:errorcluster)  [unwired: 6 in, 7 out]
      }
      frame "Set Workspace Data" {
        n27 = call "Strain Measurement.vi"("Function"=Strain_Measurement_Function."Set Workspace Data", "error in (no error)"=w76) -> ("error out"=w79:errorcluster)  [unwired: 6 in, 7 out]
      }
      frame "Set Strain Sequence Step" {
        n28 = call "Strain Measurement.vi"("Function"=Strain_Measurement_Function."Set Strain Sequence Step", "error in (no error)"=w82) -> ("error out"=w80:errorcluster)  [unwired: 6 in, 7 out]
      }
      frame "Update Sequence Status" {
        n29 = call "Strain Measurement.vi"("Function"=Strain_Measurement_Function."Update Sequence Status", "error in (no error)"=w87) -> ("error out"=w86:errorcluster)  [unwired: 6 in, 7 out]
      }
      frame "Configure Stress Control" {
        n30 = call "Strain Measurement.vi"("Function"=Strain_Measurement_Function."Configure Stress Control", "error in (no error)"=w91) -> ("error out"=w90:errorcluster)  [unwired: 6 in, 7 out]
      }
      frame "Measure Instrument Sequence" {
        n31 = call "Strain Measurement.vi"("Function"=Strain_Measurement_Function."Measure Instrument Sequence", "error in (no error)"=w95) -> ("error out"=w94:errorcluster)  [unwired: 6 in, 7 out]
      }
      frame "Save to Workspace" {
        n32 = call "Strain Measurement.vi"("Function"=Strain_Measurement_Function."Save to Workspace", "error in (no error)"=w102) -> ("error out"=w99:errorcluster)  [unwired: 6 in, 7 out]
        n33 = call "Update Status.vi"("error in"=w99, "String"="Strain Measurement Saved", "Message Queues out"=w100) -> ("error out"=w98:errorcluster)  [unwired: 8 out]
      }
      frame "Choose What Next" {
        n34 = call "Strain Measurement.vi"("Function"=Strain_Measurement_Function."Choose What Next", "error in (no error)"=w105) -> ("error out"=w106:errorcluster)  [unwired: 6 in, 7 out]
      }
      frame "Initialize" {
        n35 = Unbundle By Name(w127) -> ("Instrument Sequence.Ready"=w116:refnum<notifier>, "Stress Control.Ready"=w115:refnum<notifier>)
        n36 = Bundle By Name(cluster=w114, "Configuration"=w112) -> (w113:T59)
        n37 = Unbundle By Name(w128) -> ("Strain Measurement"=w110:refnum<queue>, "Message Handler Loop"=w123:refnum<queue>)
        n38 = call "Enqueue Message (Single).vi"("error in (no error)"=w126, "Message"="Strain Measurement - Update Refnums", "Message Queue"=w123) -> ("error out"=w124:errorcluster)  [unwired: 1 in, 7 out]
        n39 = Unbundle By Name(w113) -> ("Configuration"=w111:T44)
        n40 = call "Enqueue Message (Single).vi"("error in (no error)"=w124, "Message Data"=w111, "Message"="Strain Measurement - Set UI", "Message Queue"=w123) -> ("error out"=w117:errorcluster)  [unwired: 7 out]
        n41 = Wait on Notification(notifier=w116, error in (no error)=w117) -> (error out=w118:errorcluster)  [unwired: 5 out]
        n42 = Wait on Notification(notifier=w115, error in (no error)=w117) -> (error out=w119:errorcluster)  [unwired: 5 out]
        n43 = Merge Errors(w118, w119) -> (w108:errorcluster)
        n44 = call-poly "Enqueue Message.vi"("error in (no error)"=w108, "Message"="Get Stress Controller Status", "Message Queue"=w110) -> ("error out"=w107:errorcluster)  [unwired: 7 in, 1 out]
        n45 = call "Enqueue Message (Single).vi"("error in (no error)"=w107, "Message Data"=w111, "Message"="Define Strain Sequence", "Message Queue"=w110) -> ("error out"=w121:errorcluster)  [unwired: 7 out]
      }
      frame "Get Stress Controller Status" {
        n46 = call "Strain Measurement.vi"("Function"=Strain_Measurement_Function."Get Stress Controller Status", "error in (no error)"=w132) -> ("error out"=w131:errorcluster)  [unwired: 6 in, 7 out]
      }
      frame "Add Instrument Sequence Step" {
        n47 = call "Strain Measurement.vi"("Function"=Strain_Measurement_Function."Add Instrument Sequence Step", "error in (no error)"=w139) -> ("error out"=w135:errorcluster)  [unwired: 6 in, 7 out]
        n48 = call "Strain Measurement.vi"("Function"=Strain_Measurement_Function."Decide on Track", "Which Program?"=w133, "error in (no error)"=w135) -> ("error out"=w134:errorcluster)  [unwired: 5 in, 7 out]
      }
      frame "Clear Instrument Sequence" {
        n49 = call "Strain Measurement.vi"("Function"=Strain_Measurement_Function."Clear Instrument Sequence", "error in (no error)"=w146) -> ("error out"=w142:errorcluster)  [unwired: 6 in, 7 out]
        n50 = call "Strain Measurement.vi"("Function"=Strain_Measurement_Function."Decide on Track", "Which Program?"=w140, "error in (no error)"=w142) -> ("error out"=w141:errorcluster)  [unwired: 5 in, 7 out]
      }
      frame "Delete Instrument Sequence Step" {
        n51 = call "Strain Measurement.vi"("Function"=Strain_Measurement_Function."Delete Instrument Sequence Step", "error in (no error)"=w153) -> ("error out"=w148:errorcluster)  [unwired: 6 in, 7 out]
        n52 = call "Strain Measurement.vi"("Function"=Strain_Measurement_Function."Decide on Track", "Which Program?"=w147, "error in (no error)"=w148) -> ("error out"=w149:errorcluster)  [unwired: 5 in, 7 out]
      }
      frame "Reset Instrument Sequence" {
        n53 = call "Strain Measurement.vi"("Function"=Strain_Measurement_Function."Reset Instrument Sequence", "error in (no error)"=w160) -> ("error out"=w156:errorcluster)  [unwired: 6 in, 7 out]
        n54 = call "Strain Measurement.vi"("Function"=Strain_Measurement_Function."Decide on Track", "Which Program?"=w154, "error in (no error)"=w156) -> ("error out"=w155:errorcluster)  [unwired: 5 in, 7 out]
      }
      frame "Load Instrument Sequence" {
        n55 = call "Strain Measurement.vi"("Function"=Strain_Measurement_Function."Load Instrument Sequence", "error in (no error)"=w167) -> ("error out"=w163:errorcluster)  [unwired: 6 in, 7 out]
        n56 = call "Strain Measurement.vi"("Function"=Strain_Measurement_Function."Decide on Track", "Which Program?"=w161, "error in (no error)"=w163) -> ("error out"=w162:errorcluster)  [unwired: 5 in, 7 out]
      }
      frame "Save Instrument Sequence" {
        n57 = call "Strain Measurement.vi"("Function"=Strain_Measurement_Function."Save Instrument Sequence", "error in (no error)"=w171) -> ("error out"=w170:errorcluster)  [unwired: 6 in, 7 out]
      }
      frame "Pause" {
        n58 = call "Strain Measurement.vi"("Function"=Strain_Measurement_Function."Pause", "error in (no error)"=w175) -> ("error out"=w174:errorcluster)  [unwired: 6 in, 7 out]
      }
      frame "Stop" {
        n59 = call "Strain Measurement.vi"("Function"=Strain_Measurement_Function."Stop", "error in (no error)"=w182) -> ("error out"=w179:errorcluster)  [unwired: 6 in, 7 out]
        n60 = call "Update Status.vi"("error in"=w179, "String"="Strain Measurement Interrupted", "Message Queues out"=w176) -> ("error out"=w178:errorcluster)  [unwired: 8 out]
      }
      frame "Error" {
        # "Clear Errors to avoid getting stuck \nin repeating this case"
        # "Add here Cases that are handled \nalready by the Message Handler Loop"
        n61 = Variant To Data(error in=w191, type=errorcluster {"status"=FALSE, "code"=0, "source"=""} ("error out"), Variant=w184) -> (data=w190:errorcluster, error out=w189:errorcluster)
        n62 = Merge Errors(w190, w189) -> (w188:errorcluster)
        n63 = Unbundle By Name(w192) -> ("Message Handler Loop"=w194:refnum<queue>)
        n64 = Unbundle By Name(w188) -> ("code"=w185:i32)
        n65 = case shown="Default" w185 {
          tunnel: w194 -> [w198]
          tunnel: w188 -> [w196]
          tunnel: [w195] -> w187
          frame Default {
            n66 = call "Enqueue Message (Single).vi"("Message Data"=w196, "Message"="Error", "Message Queue"=w198) -> ("error out"=w195:errorcluster)  [unwired: 1 in, 7 out]
          }
        }
        n67 = call <vilib>:"Clear Errors.vi"("error in (no error)"=w187) -> ("error out"=w186:errorcluster)  [unwired: 1 in, 5 out]
      }
      frame "Exit" {
        w204 = TRUE ("Priority Message? (F)")
        # "Stip the VI"
        n68 = Unbundle By Name(w209) -> ("Strain Measurement"=w210:refnum<queue>)
        n69 = Release Queue(queue=w210, error in (no error)=w206) -> (error out=w199:errorcluster)  [unwired: 3 out]
        n70 = Unbundle By Name(w201) -> ("Strain Measurement.Exit"=w205:refnum<notifier>, "Strain Measurement.Ready"=w202:refnum<notifier>)
        n71 = Send Notification(notification=w204, notifier=w202, error in (no error)=w199) -> (error out=w203:errorcluster)  [unwired: 1 out]
        n72 = Send Notification(notification=w204, notifier=w205, error in (no error)=w203) -> (error out=w200:errorcluster)  [unwired: 1 out]
      }
    }
    n73 = call "Message Handling Loop.vi"("error in (no error)"=w15, "Message Queue"=w13) -> ("dup error in"=w14:errorcluster)  [unwired: 9 out]
  }
  "error out" <- w4
